vi "Manual Zero.vi"(4 "Zero":bool, 8 "error in":errorcluster, 11 "Vin":dbl[](array[numeric])) -> (0 "error out":errorcluster)   [LabVIEW 2018]
panel:
  out "New Offsets":dbl[](array[numeric])
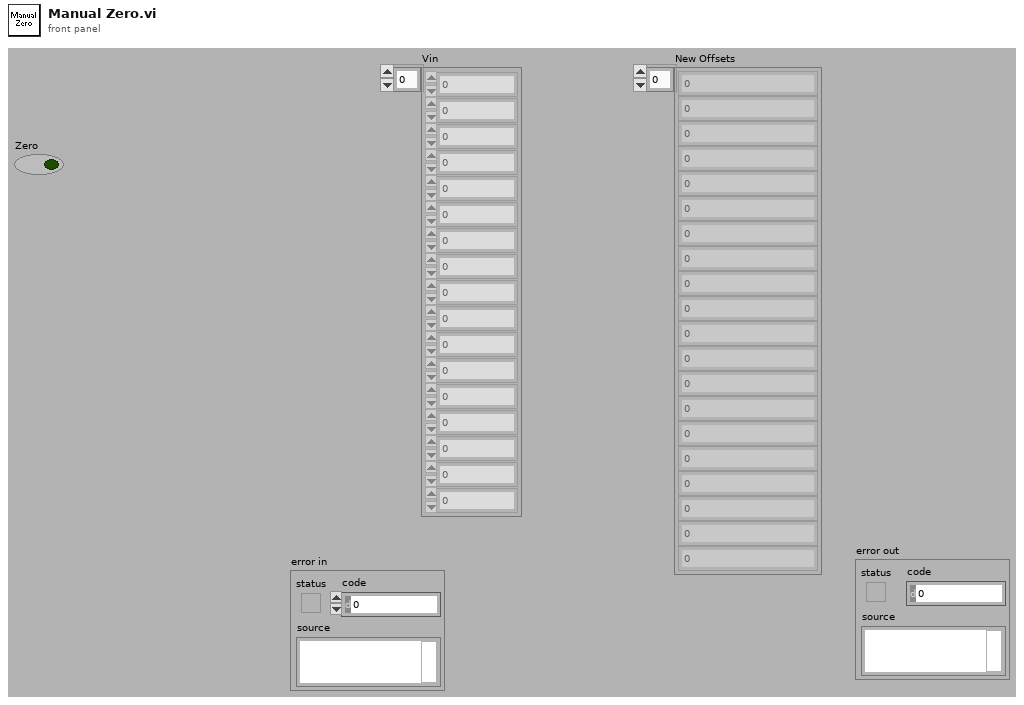
[diagram p1: front panel]
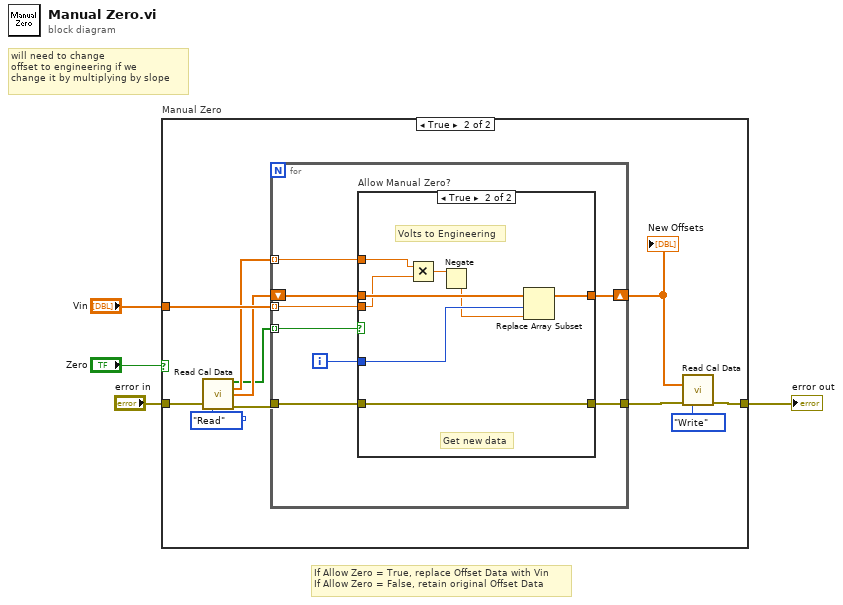
[diagram p0: block diagram]
diagram:
  # "will need to change\noffset to engineering if we\nchange it by multiplying by slope"
  # "If Allow Zero = True, replace Offset Data with Vin\nIf Allow Zero = False, retain original Offset Data"
  n1 = case "Manual Zero" shown="True" "Zero" {
    tunnel: "Vin" -> [_ w16]
    tunnel: "error in" -> [w5 w11]
    tunnel: [w5 w13] -> w4
    frame False {
    }
    frame True {
      n2 = call "Read Cal Data.vi"("error in (no error)"=w11, "Enum"=enum16{"Init", "Read", "Write"}."Read") -> ("AllowZero"=w6:bool[], "Slope"=w9:dbl[], "Offset"=w8:dbl[], "error out"=w10:errorcluster)  [unwired: 1 in, 9 out]
      n3 = for {
        tunnel: w6 -> [w18] mode=indexing
        tunnel: w16 -> [w21] mode=indexing
        shift-right: [w20] -> w15
        shift-left: w8 -> [w22]
        tunnel: w10 -> [w24]
        tunnel: [w19] -> w14
        tunnel: w9 -> [w17] mode=indexing
        i -> [w23]
        n4 = case "Allow Manual Zero?" shown="True" w18 {
          tunnel: w23 -> [_ w34]
          tunnel: [w26 w33] -> w20
          tunnel: w22 -> [w26 w32]
          tunnel: w21 -> [_ w30]
          tunnel: w24 -> [w25 w31]
          tunnel: [w25 w31] -> w19
          tunnel: w17 -> [_ w29]
          frame False {
            # "Use original data"
          }
          frame True {
            # "Volts to Engineering"
            # "Get new data"
            n5 = Multiply(x=w29, y=w30) -> (x*y=w28:dbl)
            n6 = Negate(x=w28) -> (-x=w27:dbl)
            n7 = Replace Array Subset(array=w32, new element=w27, index=w34) -> (w33:dbl[])
          }
        }
      }
      "New Offsets" <- w15
      n8 = call "Read Cal Data.vi"("NewOffsets(V)"=w15, "error in (no error)"=w14, "Enum"=enum16{"Init", "Read", "Write"}."Write") -> ("error out"=w13:errorcluster)  [unwired: 12 out]
    }
  }
  "error out" <- w4
